vi "get_counter_settings.vi"(8 "error in (no error)":errorcluster, 11 "GenericSignalWriter in":refnum<class "GenericSignalWriter.lvclass">) -> (0 "error out":errorcluster, 1 "low ticks":i32, 2 "high ticks":i32, 3 "GenericSignalWriter out":refnum<class "GenericSignalWriter.lvclass">, 4 "offset ticks":i32, 6 "counter":T1)   [LabVIEW 2010, in "GenericSignalWriter.lvclass"]
uses:
  GenericSignalWriter.lvclass
  common/clusters/counter_settings_cluster.ctl
  GenericSignalWriter.lvclass/GenericSignalWriter.ctl
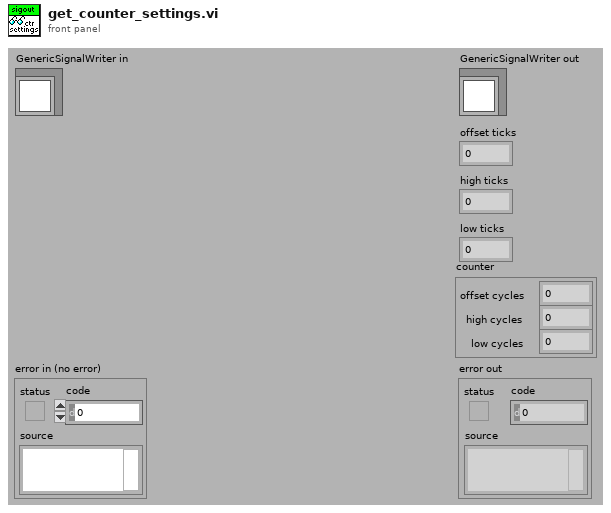
[diagram p1: front panel]
types:
  T1 = typedef "counter_settings_cluster.ctl" = cluster{"offset cycles":i32, "high cycles":i32, "low cycles":i32}
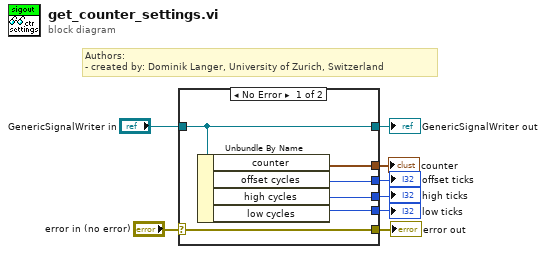
[diagram p0: block diagram]
diagram:
  # "Authors: \n- created by: Dominik Langer, University of Zurich, Switzerland"
  n1 = case shown="No Error" "error in (no error)" {
    selector: "error in (no error)" -> [w14 w16]
    tunnel: [w14 w16] -> w7
    tunnel: [w13 w15] -> w5
    tunnel: "GenericSignalWriter in" -> [w13 w15]
    tunnel: [w12 _] -> w2
    tunnel: [w11 _] -> w3
    tunnel: [w10 _] -> w4
    tunnel: [w9 _] -> w1
    frame No Error {
      n2 = Unbundle By Name(w13) -> ("counter"=w9:T1, "offset cycles"=w12:i32, "high cycles"=w11:i32, "low cycles"=w10:i32)
    }
    frame Error {
    }
  }
  "error out" <- w7
  "GenericSignalWriter out" <- w5
  "offset ticks" <- w2
  "high ticks" <- w3
  "low ticks" <- w4
  "counter" <- w1
